vi "USBData_initialize_dummy.vi"(0 "USBData in":refnum<class "USBData.lvclass">, 1 "Activate?":bool=TRUE, 3 "RUN start time":timestamp, 5 "BasePath":path, 7 "RunName":string, 9 "InstName":string, 11 "error in (no error)":errorcluster, 12 "SeriesSetting":T1(array[cluster])) -> (2 "Labels(indicator)":string[](array[string]), 4 "USBData out":refnum<class "USBData.lvclass">, 6 "FileFormatLD":string, 8 "LabelLD":string, 10 "LeakDetetcorRead?":bool=TRUE, 14 "Status":T2(ring), 15 "error out":errorcluster)   [LabVIEW 2017, in "USBData.lvclass"]
uses:
  USBData.lvclass
  USBData.lvclass/USBData.ctl
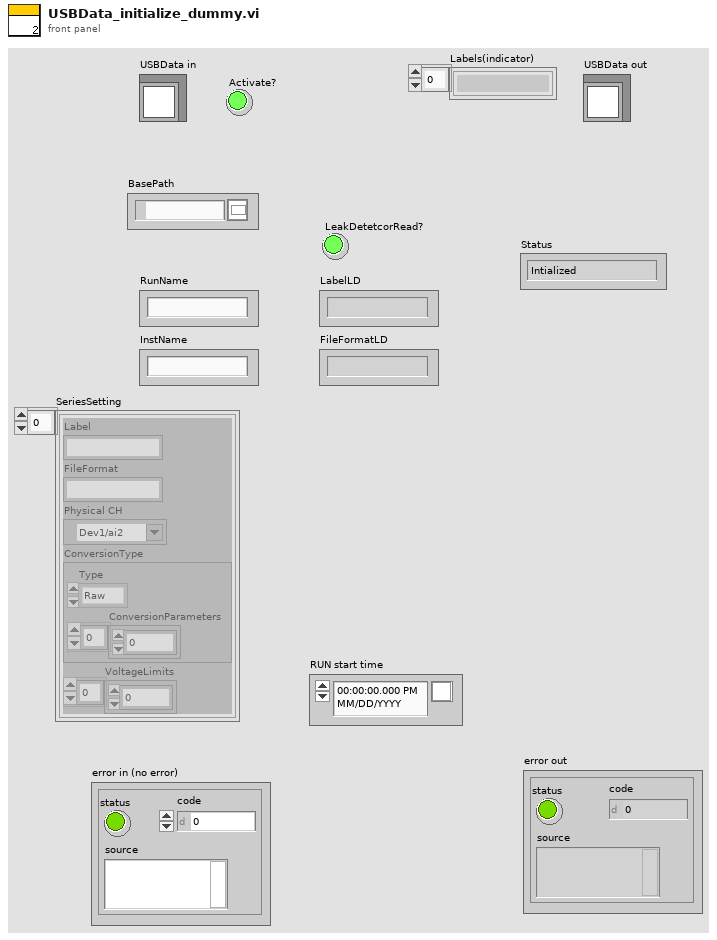
[diagram p1: front panel]
types:
  T1 = cluster{"Label":string, "FileFormat":string, "Physical CH":tag, "ConversionType":cluster{"Type":enum16{"Raw", "SimpleProp", "CC-10_COMBINED", "CC-10_LOG", "LeakDet_EXP", "LeakDet_Mantissa", "Baratron"}, "ConversionParameters":dbl[]}, "VoltageLimits":dbl[]}[]
  T2 = enum16{"Intialized", "Waiting", "Measuring", "Terminated"}
  T3 = cluster{"Type":enum16{"SimpleProp", "CC-10_COMBINED", "CC-10_LOG", "LeakDet_EXP", "LeakDet_Mantissa", "Baratron"}, "ConversionParameters":dbl[]}[]
  T4 = enum16{"SimpleProp", "CC-10_COMBINED", "CC-10_LOG", "LeakDet_EXP", "LeakDet_Mantissa", "LeakDet_Full"}
  T5 = cluster{"Type":enum16{"Raw", "SimpleProp", "CC-10_COMBINED", "CC-10_LOG", "LeakDet_EXP", "LeakDet_Mantissa", "Baratron"}, "ConversionParameters":dbl[]}
  T6 = enum16{"Raw", "SimpleProp", "CC-10_COMBINED", "CC-10_LOG", "LeakDet_EXP", "LeakDet_Mantissa", "Baratron"}
  T7 = cluster{"Type":u16, "ConversionParameters":dbl[]}[]
  T8 = enum16{"open", "replace", "create", "open or create", "replace or create", "replace or create with confirmation"}
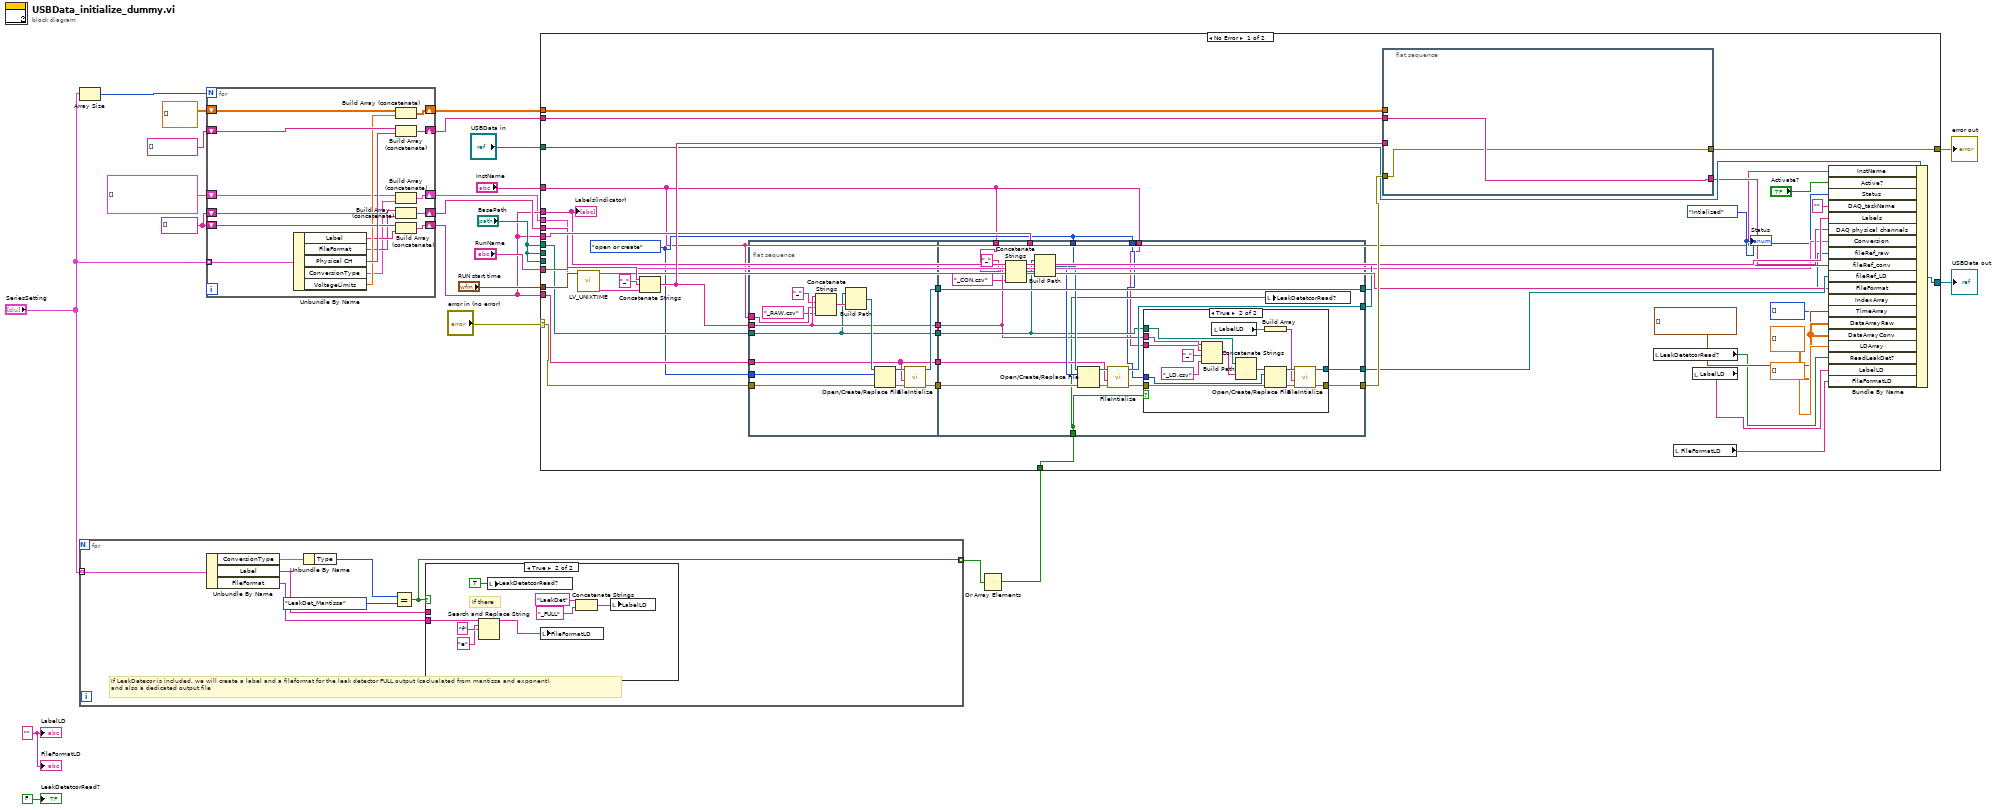
[diagram p0: block diagram]
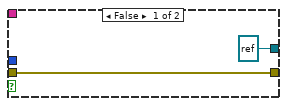
[diagram p3: hidden frame]
diagram:
  w13 = "" ("LabelLD")
  w18 = string[] []
  n1 = Array Size(array="SeriesSetting") -> (size(s)=w6:i32)
  n2 = for {
    tunnel: "SeriesSetting" -> [w30] mode=indexing
    tunnel: [w24] -> w3 mode=indexing
    # "If LeakDetecor is included, we will create a label and a fileformat for the leak detector FULL output (caclualated from mantissa and exponent), \nand also a dedicated output file"
    n3 = Unbundle By Name(w30) -> ("ConversionType"=w29:T5, "Label"=w26:string, "FileFormat"=w25:string)
    n4 = Unbundle By Name(w29) -> ("Type"=w28:T6)
    n5 = Equal?(x=w28, y=T4."LeakDet_Mantissa") -> (x = y?=w24:bool)
    n6 = case shown="True" w24 {
      tunnel: w26 -> [_ _]
      tunnel: w25 -> [_ w32]
      frame False {
      }
      frame True {
        # "If there"
        n7 = Search and Replace String(input string=w32, search string="f", replace string="e" ("replace string (\"\")")) -> (result string=w35:string)  [unwired: 5 in, 3 out]
        n8 = local write "LeakDetetcorRead?"(TRUE ("LeakDetetcorRead?")) -> ()
        n9 = local write "FileFormatLD"(w35) -> ()
        n10 = Concatenate Strings("LaekDet" ("string"), "_FULL" ("string")) -> (w33:string)
        n11 = local write "LabelLD"(w33) -> ()
      }
    }
  }
  n12 = for {
    N: w6 -> [_]
    tunnel: "SeriesSetting" -> [w54] mode=indexing
    shift-right: [w52] -> w10
    shift-left: tag[] [] -> [w47]
    shift-right: [w51] -> w7
    shift-left: w18 -> [w50]
    shift-right: [w49] -> w9
    shift-left: w18 -> [w48]
    shift-right: [w45] -> w11
    shift-left: dbl[][] [] -> [w44]
    shift-right: [w40] -> w5
    shift-left: T3 [] ("Conversion") -> [w39]
    n13 = Unbundle By Name(w54) -> ("Label"=w43:string, "FileFormat"=w42:string, "Physical CH"=w53:tag, "ConversionType"=w41:T5, "VoltageLimits"=w46:dbl[])
    n14 = Build Array (concatenate)(w44, w46) -> (w45:dbl[][])
    n15 = Build Array (concatenate)(w47, w53) -> (w52:tag[])
    n16 = Build Array (concatenate)(w39, w41) -> (w40:T7)
    n17 = Build Array (concatenate)(w48, w42) -> (w49:string[])
    n18 = Build Array (concatenate)(w50, w43) -> (w51:string[])
  }
  n19 = Or Array Elements(Boolean array=w3) -> (logical OR=w2:bool)
  n20 = case shown="No Error" "error in (no error)" {
    selector: "error in (no error)" -> [w87 w149]
    tunnel: [w55 w149] -> w22
    tunnel: "USBData in" -> [w77 w148]
    tunnel: [w66 w148] -> w20
    tunnel: w10 -> [w90 _]
    tunnel: "InstName" -> [w57 _]
    tunnel: w7 -> [w75 _]
    tunnel: w9 -> [w69 _]
    tunnel: "BasePath" -> [_ _]
    tunnel: "RunName" -> [w93 _]
    tunnel: "RUN start time" -> [w92 _]
    tunnel: w11 -> [w89 _]
    tunnel: "BasePath" -> [w88 _]
    tunnel: w7 -> [w86 _]
    tunnel: "BasePath" -> [_ _]
    tunnel: w7 -> [w82 _]
    tunnel: w5 -> [w64 _]
    tunnel: w2 -> [w60 _]
    frame No Error {
      w59 = T8."open or create" ("operation (0:open)")
      w72 = dbl[][] [] ("DataArray")
      w58 = T2."Intialized" ("Status")
      n21 = call "LV_UNIXTIME.vi"("current time"=w92) -> ("date/time string"=w94:string)  [unwired: 9 in, 1 out]
      n22 = Concatenate Strings(w93, "_" ("string"), w94) -> (w83:string)
      n23 = flat-sequence {
        tunnel: w83 -> [w99]
        tunnel: w88 -> [w98]
        tunnel: w87 -> [w107]
        tunnel: w59 -> [w106]
        tunnel: w86 -> [w100]
        tunnel: [w102] -> w85
        tunnel: [w101] -> w84
        tunnel: [w100] -> w81
        tunnel: [w99] -> w80
        tunnel: [w98] -> w79
        tunnel: w57 -> [w96]
        tunnel: [w128] -> w67
        tunnel: w85 -> [w126]
        tunnel: w84 -> [w128]
        tunnel: w59 -> [w125]
        tunnel: w82 -> [_]
        tunnel: [w121] -> w68
        tunnel: w81 -> [w120]
        tunnel: w80 -> [w118]
        tunnel: w79 -> [w119]
        tunnel: [w116] -> w78
        tunnel: [w115] -> w74
        tunnel: w60 -> [w114]
        tunnel: w59 -> [w113]
        tunnel: w57 -> [w112]
        tunnel: w57 -> [w109]
        frame #0 {
          n24 = Concatenate Strings(w99, "_" ("string"), w96, "_RAW.csv" ("string")) -> (w108:string)
          n25 = Build Path(base path=w98, name or relative path=w108) -> (appended path=w105:path)
          n26 = Open/Create/Replace File(file path (use dialog)=w105, error in=w107, operation (0:open)=w106) -> (refnum out=w103:refnum<file>, error out=w104:errorcluster)  [unwired: 3 in, 1 out]
          n27 = call "FileIntialize.vi"("Error In"=w104, "Labels"=w100, "refnum in"=w103) -> ("Error Out"=w102:errorcluster, "File Refnum"=w101:refnum<file>)  [unwired: 7 in]
        }
        frame #1 {
          n28 = Concatenate Strings(w118, w112, "_" ("string"), "_CON.csv" ("string")) -> (w127:string)
          n29 = Build Path(base path=w119, name or relative path=w127) -> (appended path=w124:path)
          n30 = Open/Create/Replace File(file path (use dialog)=w124, error in=w126, operation (0:open)=w125) -> (refnum out=w122:refnum<file>, error out=w123:errorcluster)  [unwired: 3 in, 1 out]
          n31 = call "FileIntialize.vi"("Error In"=w123, "Labels"=w120, "refnum in"=w122) -> ("Error Out"=w117:errorcluster, "File Refnum"=w121:refnum<file>)  [unwired: 7 in]
          n32 = case shown="True" w114 {
            tunnel: w119 -> [_ w143]
            tunnel: w118 -> [_ w142]
            tunnel: w117 -> [w130 w137]
            tunnel: [w130 w136] -> w116
            tunnel: [refnum<file> refnum ("File Refnum") w135] -> w115
            tunnel: w113 -> [_ w134]
            tunnel: w109 -> [_ w131]
            frame False {
            }
            frame True {
              n33 = Concatenate Strings(w142, w131, "_" ("string"), "_LD.csv" ("string")) -> (w144:string)
              n34 = local read "LabelLD"() -> (w139:string)
              n35 = Build Path(base path=w143, name or relative path=w144) -> (appended path=w140:path)
              n36 = Build Array(w139) -> (w138:string[])
              n37 = Open/Create/Replace File(file path (use dialog)=w140, error in=w137, operation (0:open)=w134) -> (refnum out=w141:refnum<file>, error out=w145:errorcluster)  [unwired: 3 in, 1 out]
              n38 = call "FileIntialize.vi"("Error In"=w145, "Labels"=w138, "refnum in"=w141) -> ("Error Out"=w136:errorcluster, "File Refnum"=w135:refnum<file>)  [unwired: 7 in]
            }
          }
          n39 = local write "LeakDetetcorRead?"(w114) -> ()
        }
      }
      n40 = flat-sequence {
        tunnel: w83 -> [_]
        tunnel: w90 -> [w147]
        tunnel: w89 -> [_]
        tunnel: w78 -> [w146]
        tunnel: [w147] -> w65
        tunnel: [w146] -> w55
        frame #0 {
        }
      }
      n41 = local read "LeakDetetcorRead?"() -> (w63:bool)
      n42 = local read "FileFormatLD"() -> (w61:string)
      n43 = local read "LabelLD"() -> (w62:string)
      n44 = Bundle By Name(cluster=w77, "InstName"=w57, "Active?"="Activate?", "Status"=w58, "DAQ_taskName"="", "Labels"=w75, "DAQ physical channels"=w65, "Conversion"=w64, "fileRef_raw"=w67, "fileRef_conv"=w68, "fileRef_LD"=w74, "FileFormat"=w69, "IndexArray"=i64[] [], "TimeArray"=timestamp[] [], "DataArrayRaw"=w72, "DataArrayConv"=w72, "LDArray"=dbl[] [], "ReadLeakDet?"=w63, "LabelLD"=w62, "FileFormatLD"=w61) -> (w66:refnum<class "USBData.lvclass">)
      "Labels(indicator)" <- w75
      "Status" <- w58
    }
    frame Error {
    }
  }
  "error out" <- w22
  "USBData out" <- w20
  "FileFormatLD" <- w13
  "LabelLD" <- w13
  "LeakDetetcorRead?" <- FALSE ("LeakDetetcorRead?")
